vi "Build Calibrate.vi"(8 "error in (no error)":errorcluster, 10 "Module.lvclass":refnum<class "Module.lvclass">, 11 "Calibrate in":refnum<class "Calibrate.lvclass">) -> (0 "error out":errorcluster, 3 "Calibrate out":refnum<class "Calibrate.lvclass">)   [LabVIEW 2020, in "Calibrate.lvclass"]
uses:
  Calibrate.lvclass
  C:/Users/HEP/Documents/Aerotech gantry/UCSB-Gantry-master-main/V5/Classes/Assembly/Assembly Run.lvclass
  Module/Module.lvclass
  Workspace/Fixture Enum.ctl
  Routine/Routine Enum.ctl
  Calibrate.lvclass/Calibrate.ctl
  Workspace/Fixture.lvclass
  Routine/Routine.lvclass
  Assembly Run.lvclass
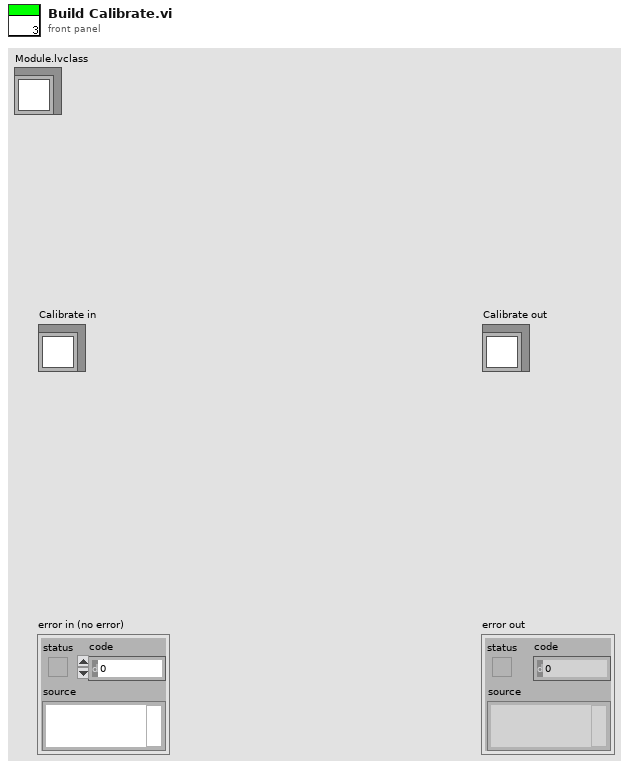
[diagram p1: front panel]
types:
  T1 = typedef "Fixture.lvclass/Fixture Enum.ctl" = enum16{"Assembly Tray", "Syringe Space", "Component", "Pick Up Tool", "Current Position"}
  T2 = typedef "Routine.lvclass/Routine Enum.ctl" = enum16{"Primary Pick Up", "Pick Up All", "Put Down Secondary", "Put Down All", "Release Syringe", "Secondary Pick Up", "Secure Syringe", "Dispense on Plate", "Dispense on Kapton", "Dispense on Sensor", "Dispense Offset"}
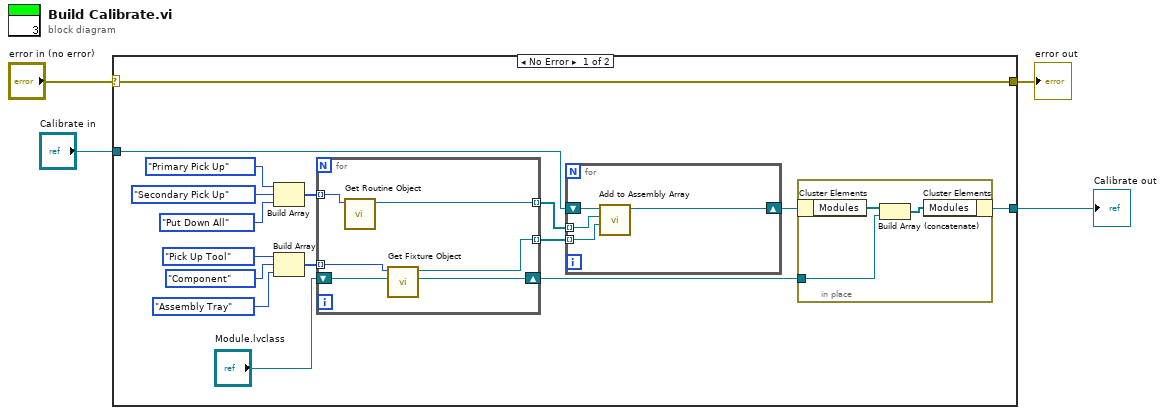
[diagram p0: block diagram]
diagram:
  n1 = case shown="No Error" "error in (no error)" {
    selector: "error in (no error)" -> [w20 w35]
    tunnel: [w20 w35] -> w3
    tunnel: [w6 w34] -> w1
    tunnel: "Calibrate in" -> [w9 w34]
    frame No Error {
      n2 = Build Array(Routine_Enum."Primary Pick Up" ("Routine"), Routine_Enum."Secondary Pick Up" ("Routine"), Routine_Enum."Put Down All" ("Routine")) -> (w18:T2[])
      n3 = Build Array(Fixture_Enum."Pick Up Tool" ("Fixture"), Fixture_Enum."Component" ("Fixture"), Fixture_Enum."Assembly Tray" ("Fixture")) -> (w19:T1[])
      n4 = for {
        tunnel: w18 -> [w33] mode=indexing
        tunnel: [w31] -> w11 mode=indexing
        tunnel: w19 -> [w32] mode=indexing
        tunnel: [w28] -> w10 mode=indexing
        shift-right: [w29] -> w8
        shift-left: "Module.lvclass" -> [w30]
        n5 = call "Get Routine Object.vi"("Routine"=w33) -> ("Routine out"=w31:refnum<class "Routine.lvclass">)  [unwired: 9 in, 1 out]
        n6 = call "Get Fixture Object.vi"("Module In"=w30, "Fixture"=w32) -> ("Module Out"=w29:refnum<class "Module.lvclass">, "Workspace.lvclass"=w28:refnum<class "Fixture.lvclass">)  [unwired: 7 in, 1 out]
      }
      n7 = for {
        tunnel: w11 -> [w27] mode=indexing
        tunnel: w10 -> [w26] mode=indexing
        shift-right: [w24] -> w7
        shift-left: w9 -> [w25]
        n8 = call "Add to Assembly Array.vi"("Workspace In"=w26, "Routine In"=w27, "Assembly Run in"=w25) -> ("Assembly Run out"=w24:refnum<class "Calibrate.lvclass">)  [unwired: 7 in, 1 out]
      }
      n9 = in-place {
        in-place-border: w8 -> [w21]
        n10 = in-place-cluster #1(w7) -> ("Modules"=w23:refnum<class "Module.lvclass">[])
        n11 = Build Array (concatenate)(w23, w21) -> (w22:refnum<class "Module.lvclass">[])
        n12 = in-place-cluster #1("Modules"=w22) -> (w6:refnum<class "Calibrate.lvclass">)
      }
    }
    frame Error {
    }
  }
  "error out" <- w3
  "Calibrate out" <- w1
